vi "ex1.vi"() -> ()   [LabVIEW 2022 SP3]
uses:
  <vilib>/numeric/Random Number (Range) DBL.vi
panel:
  in  "Noises Amplitude":dbl
  out "Waveform Chart":dbl(graph)
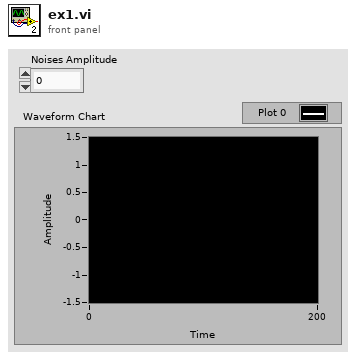
[diagram p1: front panel]
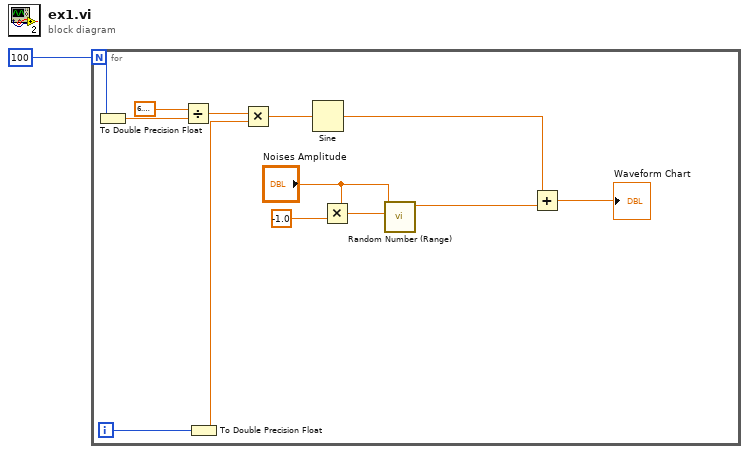
[diagram p0: block diagram]
diagram:
  n1 = for {
    N: 100 -> [w8]
    i -> [w11]
    n2 = To Double Precision Float(number=w8) -> (double precision float=w9:dbl)
    n3 = Divide(x=6.283185307179586, y=w9) -> (x/y=w13:dbl)
    n4 = To Double Precision Float(number=w11) -> (double precision float=w10:dbl)
    n5 = Multiply(x=w13, y=w10) -> (x*y=w12:dbl)
    n6 = Sine(x=w12) -> (sin(x)=w4:dbl)
    n7 = Multiply(x="Noises Amplitude", y=-1.0) -> (x*y=w6:dbl)
    n8 = call-poly <vilib>:"Random Number (Range).vi"("lower bound (0)"=w6, "upper bound (100)"="Noises Amplitude") -> ("number"=w3:dbl)  [unwired: 9 in]
    n9 = Add(x=w4, y=w3) -> (x+y=→"Waveform Chart":dbl)
  }
